vi "Read Digital IO Data.vi"(8 "error in (no error)":errorcluster, 9 "Digital Line (1)":i32=1, 10 "Data Type (0: Bit)":i32(ring) items=["Bit", "Port"], 11 "VISA resource name":refnum<visa-resource-name>) -> (0 "error out":errorcluster, 1 "Port":i32, 2 "Bit":i32, 3 "VISA resource name out":refnum<visa-resource-name>)   [LabVIEW 2019, in "Keithley 2600 Series.lvlib"]
doc: "Returns data from the digital IO lines.\n\n<b>Note:</b>\nThis VI is not available on the models 2604B, 2614B, and 2634B."
uses:
  Keithley 2600 Series.lvlib
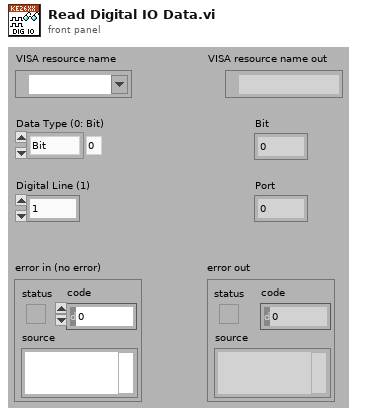
[diagram p1: front panel]
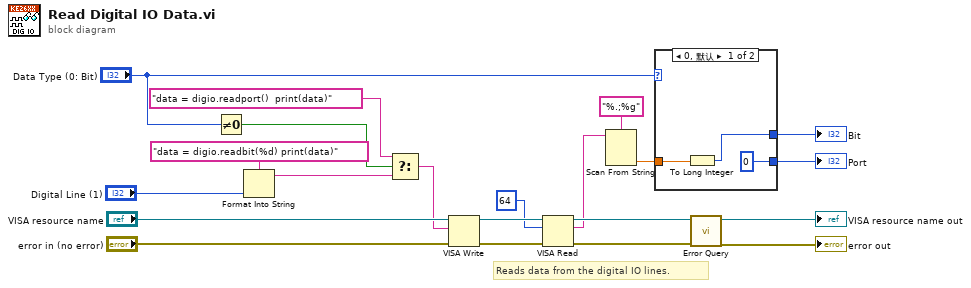
[diagram p0: block diagram]
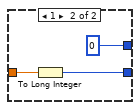
[diagram p2: hidden frame]
diagram:
  # "Reads data from the digital IO lines."
  n1 = Not Equal To 0?(x="Data Type (0: Bit)") -> (x != 0?=w7:bool)
  n2 = Format Into String(format string="data = digio.readbit(%d) print(data)", "Digital Line (1)") -> (resulting string=w4:string)  [unwired: 2 in, 1 out]
  n3 = Select(t="data = digio.readport()  print(data)", s=w7, f=w4) -> (s? t:f=w3:string)
  n4 = VISA Write(VISA resource name="VISA resource name", write buffer=w3, error in (no error)="error in (no error)") -> (VISA resource name out=w17:refnum<visa-resource-name>, error out=w16:errorcluster)  [unwired: 1 out]
  n5 = VISA Read(VISA resource name=w17, byte count=u32 64, error in (no error)=w16) -> (VISA resource name out=w15:refnum<visa-resource-name>, read buffer=w12:string, error out=w14:errorcluster)  [unwired: 1 out]
  n6 = Scan From String(format string="%.;%g", input string=w12) -> (output 1=w10:dbl)  [unwired: 3 in, 3 out]
  n7 = case shown="0, 默认" "Data Type (0: Bit)" {
    tunnel: w10 -> [w24 w27]
    tunnel: [w23 0] -> w2
    tunnel: [0 w26] -> w1
    frame 0, Default {
      n8 = To Long Integer(number=w24) -> (32bit integer=w23:i32)
    }
    frame 1 {
      n9 = To Long Integer(number=w27) -> (32bit integer=w26:i32)
    }
  }
  "Bit" <- w2
  "Port" <- w1
  n10 = call "Error Query.vi"("error in (no error)"=w14, "VISA resource name"=w15) -> ("error out"=→"error out":errorcluster, "VISA resource name out"=→"VISA resource name out":refnum<visa-resource-name>)  [unwired: 6 in, 2 out]
